vi "日志、报警信息存储 (子VI).vi"() -> ()   [LabVIEW 2016, in "超标留样集成.lvlib" / "德润DR803M超标留样.lvlib"]
uses:
  <vilib>/ptbypt/NI_PtbyPt.lvlib
panel:
  out "MB仪器状态":T1 {"当前进程" items=["停止中"=0, "启动延时"=1, "外置泵延时"=2, "管路润洗"=3, "管存"=4, "留样"=5, "出水管路排空"=6, "采水管路排空"=7, "瓶位调整"=12, "待机"=13]; "工作模式" items=["定时留样"=1, "时间等比"=2, "同步留样"=3, "外控留样"=4, "超标留样"=5]; "仪器时间" format="%<%Y/%m/%d %H:%M:%S>T"}
  out "仪器状态":T2 {"仪器时间" format="%<%Y/%m/%d %H:%M:%S>T"; "门状态" items=["关闭", "打开"]; "采样模式" items=["定时留样"=1, "时间等比"=2, "同步留样"=3, "外控留样"=4, "超标留样"=5]; "工作进程" items=["停止中"=0, "启动延时"=1, "外置泵延时"=2, "管路润洗"=3, "管存"=4, "留样"=5, "出水管路排空"=6, "采水管路排空"=7, "待机"=13]; "工作状态" items=["停止", "运行", "系统初始化"]}
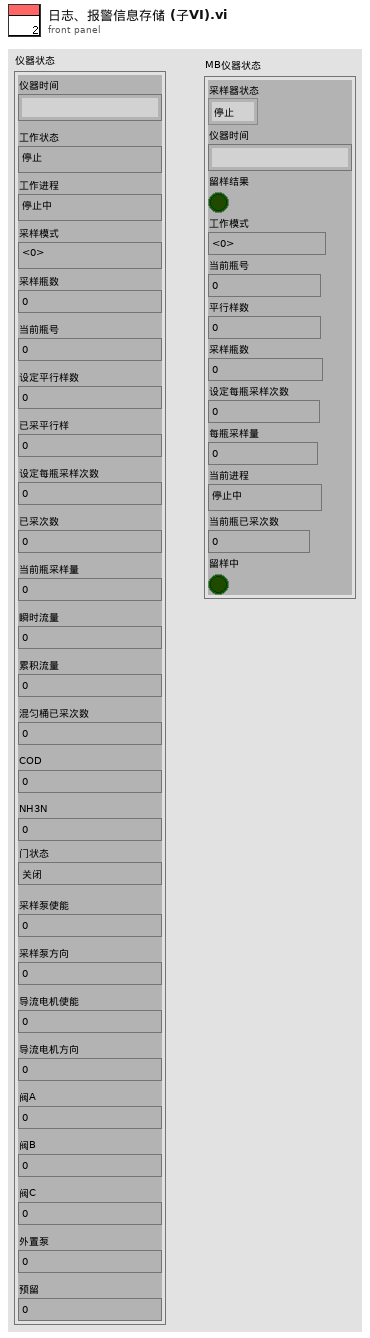
[diagram p1: front panel]
types:
  T1 = cluster{"采样器状态":enum16{"停止", "运行", "系统初始化-2", "系统初始化-3", "初始化失败"}, "仪器时间":timestamp, "留样结果":bool, "工作模式":u16, "当前瓶号":u16, "平行样数":u16, "采样瓶数":u16, "设定每瓶采样次数":u16, "每瓶采样量":u16, "当前进程":u16, "当前瓶已采次数":u16, "留样中":bool}
  T2 = cluster{"仪器时间":timestamp, "工作状态":u16, "工作进程":u16, "采样模式":u16, "采样瓶数":dbl, "当前瓶号":dbl, "设定平行样数":dbl, "已采平行样":dbl, "设定每瓶采样次数":dbl, "已采次数":dbl, "当前瓶采样量":dbl, "瞬时流量":dbl, "累积流量":dbl, "混匀桶已采次数":dbl, "COD":dbl, "NH3N":dbl, "门状态":u16, "采样泵使能":dbl, "采样泵方向":dbl, "导流电机使能":dbl, "导流电机方向":dbl, "阀A":dbl, "阀B":dbl, "阀C":dbl, "外置泵":dbl, "预留":dbl}
  T3 = cluster{"时间标识":timestamp, "设备":string, "日志信息":string}
  T4 = cluster{"时间标识":timestamp, "设备":string, "日志信息":string, "流程参数":string}
  T5 = enum16{"停止", "运行", "系统初始化-2", "系统初始化-3", "初始化失败"}
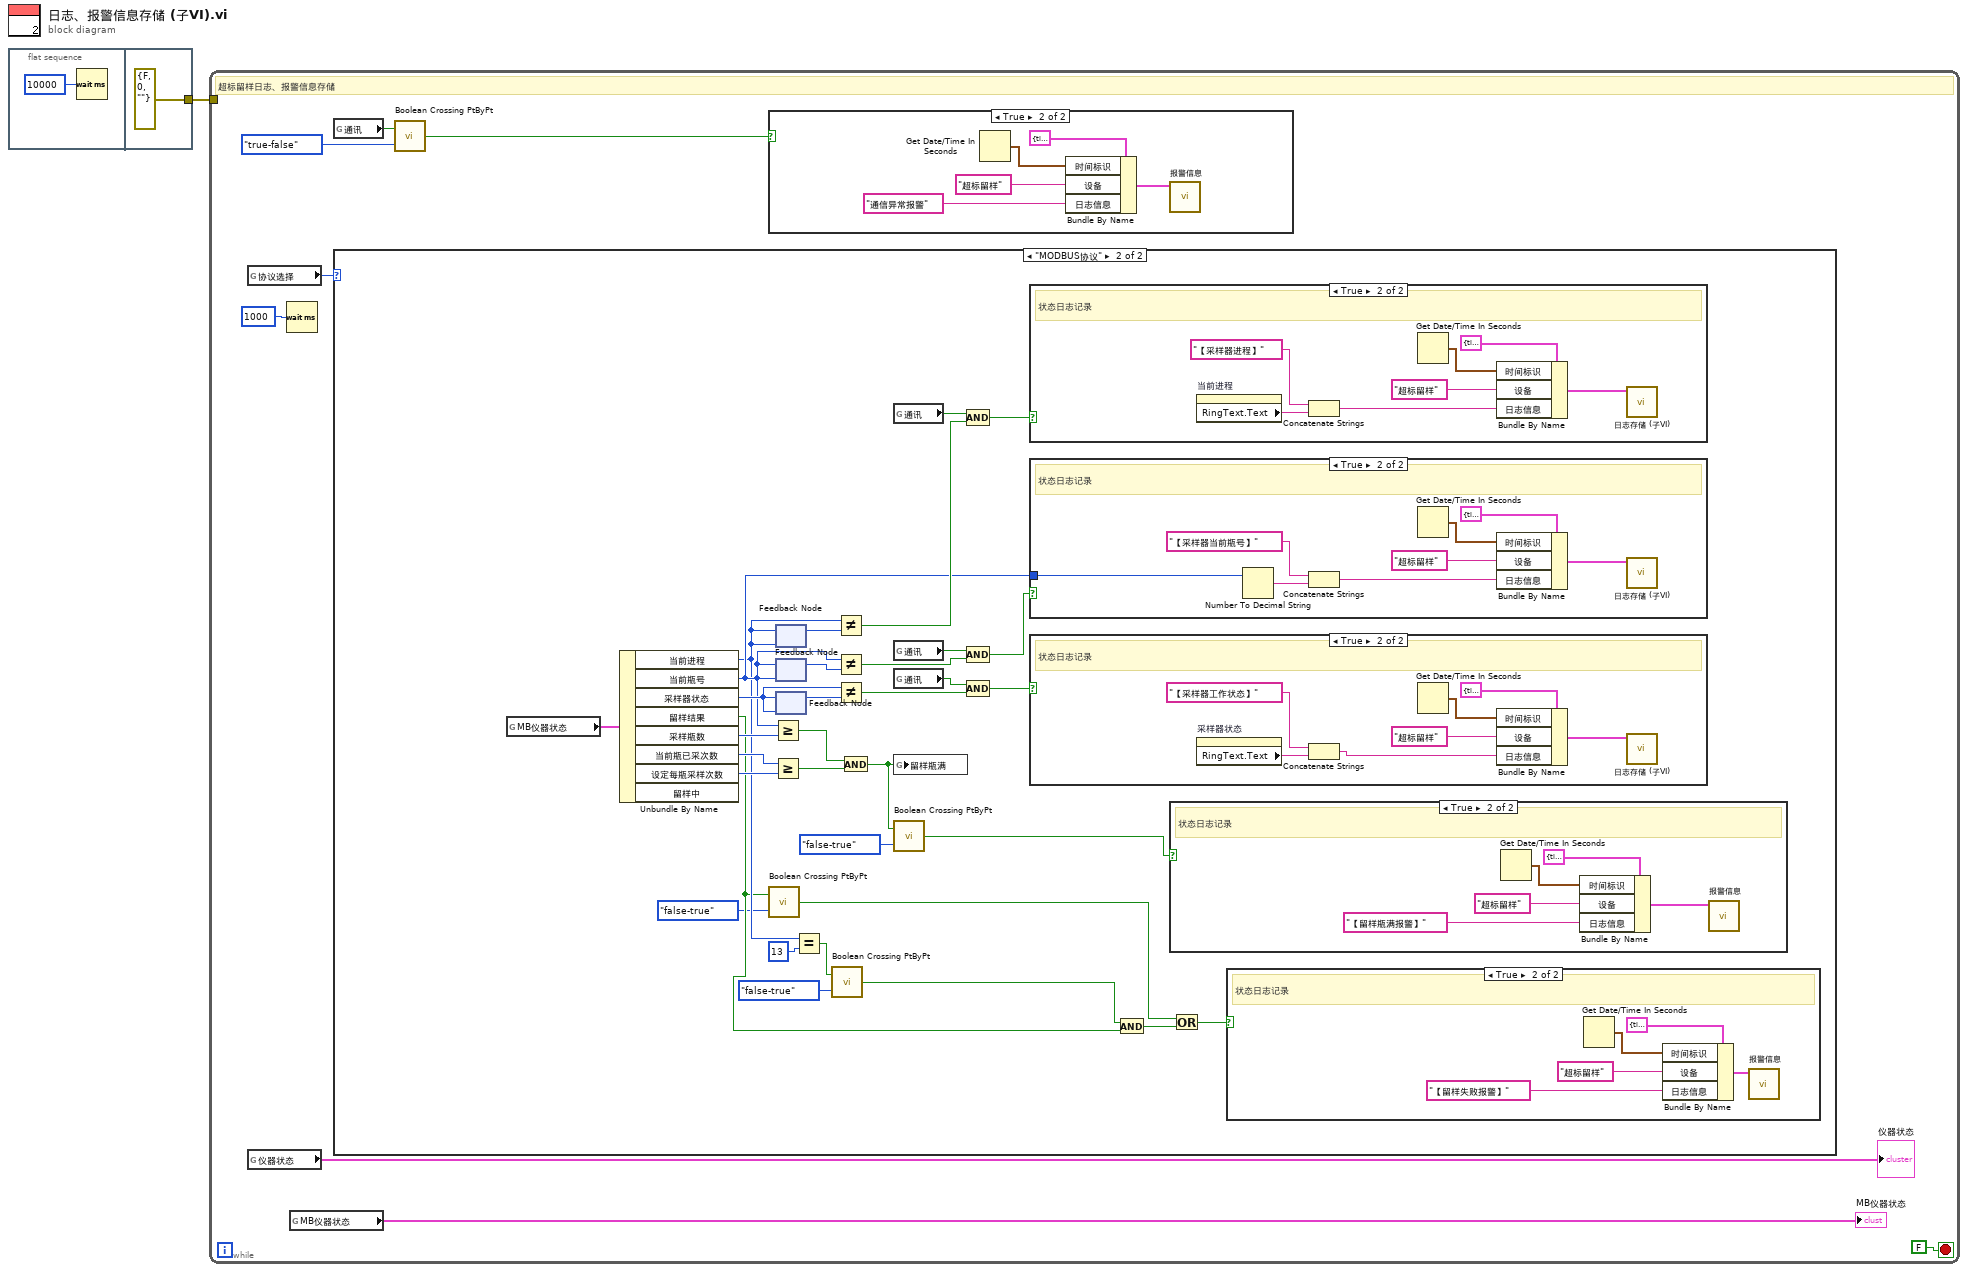
[diagram p0: block diagram]
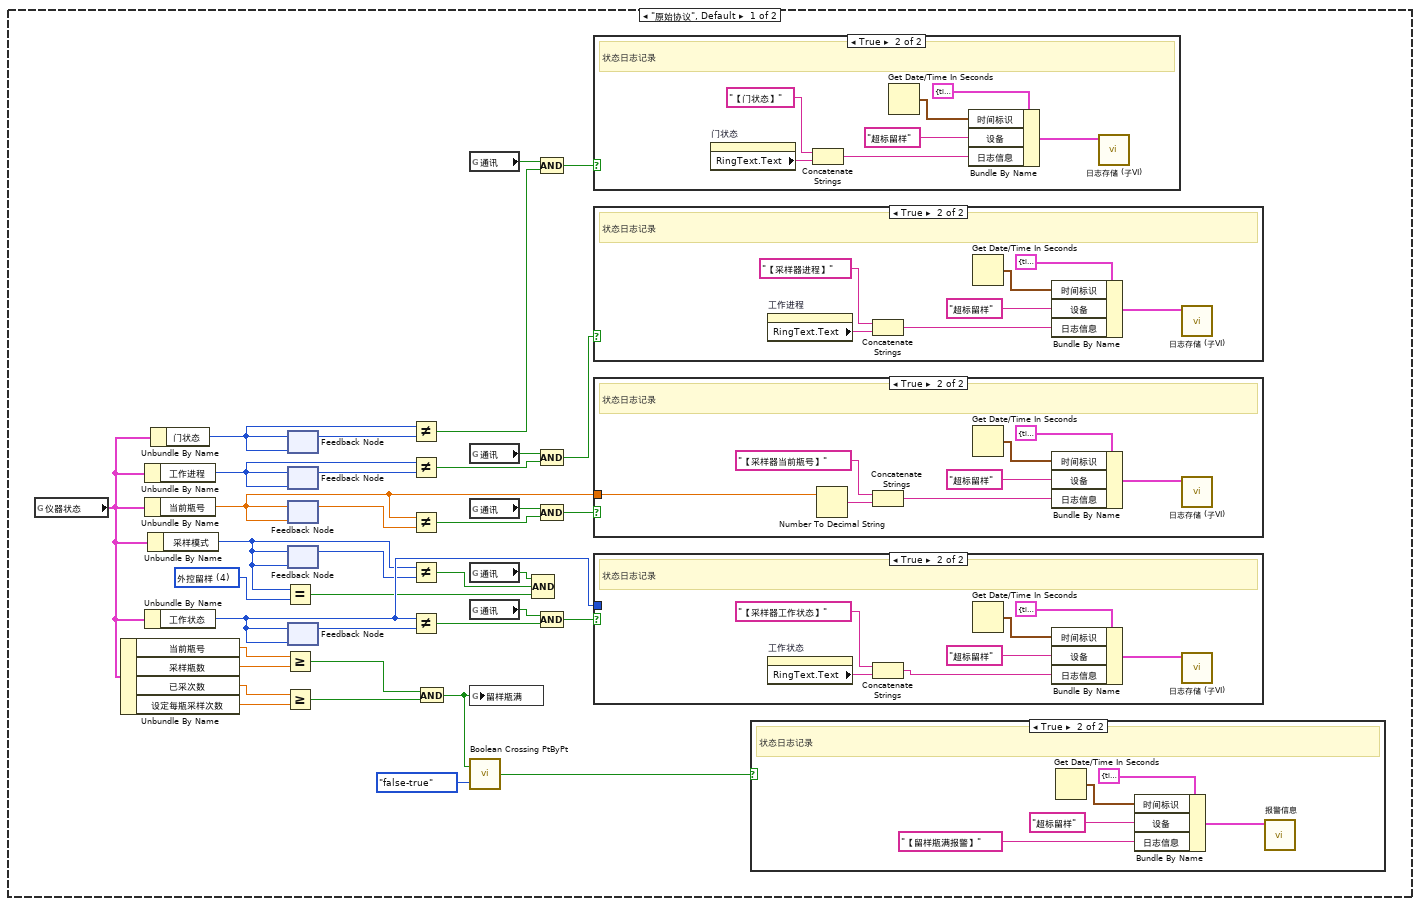
[diagram p2: hidden frame]
diagram:
  n1 = flat-sequence {
    tunnel: [errorcluster {"status"=FALSE, "code"=0, "source"=""} ("错误常量")] -> w1
    frame #0 {
      n2 = Wait (ms)(milliseconds to wait=u32 10000 ("等待时间（毫秒）")) -> ()  [unwired: 1 out]
    }
    frame #1 {
    }
  }
  n3 = while {
    tunnel: w1 -> [_]
    stop <- FALSE stop-if-true
    # "超标留样日志、报警信息存储"
    n4 = global read "超标留样全局.vi" "协议选择"() -> (w6:enum16{"原始协议", "MODBUS协议"})
    n5 = global read "超标留样全局.vi" "仪器状态"() -> (→"仪器状态":T2)
    n6 = Wait (ms)(milliseconds to wait=u32 1000 ("等待时间（毫秒）")) -> ()  [unwired: 1 out]
    n7 = global read "超标留样全局.vi" "MB仪器状态"() -> (→"MB仪器状态":T1)
    n8 = global read "超标留样全局.vi" "通讯"() -> (w7:bool)
    n9 = case shown="\"MODBUS协议\"" w6 {
      frame "原始协议", Default {
        w23 = u16 4 items=["定时留样"=1, "时间等比"=2, "同步留样"=3, "外控留样"=4, "超标留样"=5] ("采样模式")
        n10 = global read "超标留样全局.vi" "仪器状态"() -> (w22:T2)
        n11 = Unbundle By Name(w22) -> ("当前瓶号"=w21:dbl, "采样瓶数"=w20:dbl, "已采次数"=w19:dbl, "设定每瓶采样次数"=w18:dbl)
        n12 = Unbundle By Name(w22) -> ("工作进程"=w47:u16)
        n13 = Unbundle By Name(w22) -> ("当前瓶号"=w44:dbl)
        n14 = Unbundle By Name(w22) -> ("工作状态"=w43:u16)
        n15 = Unbundle By Name(w22) -> ("采样模式"=w39:u16)
        n16 = Unbundle By Name(w22) -> ("门状态"=w40:u16)
        n17 = Equal?(x=w39, y=w23) -> (x = y?=w25:bool)
        n18 = Greater Or Equal?(x=w21, y=w20) -> (x >= y?=w17:bool)
        n19 = Greater Or Equal?(x=w19, y=w18) -> (x >= y?=w16:bool)
        n20 = feedback #1(w40) -> (w41:u16)
        n21 = feedback-in #1(w40) -> ()
        n22 = feedback #2(w47) -> (w46:u16)
        n23 = feedback-in #2(w47) -> ()
        n24 = feedback #3(w44) -> (w45:dbl)
        n25 = feedback-in #3(w44) -> ()
        n26 = feedback #4(w39) -> (w38:u16)
        n27 = feedback-in #4(w39) -> ()
        n28 = feedback #5(w43) -> (w42:u16)
        n29 = feedback-in #5(w43) -> ()
        n30 = Not Equal?(x=w40, y=w41) -> (x != y?=w35:bool)
        n31 = Not Equal?(x=w47, y=w46) -> (x != y?=w33:bool)
        n32 = Not Equal?(x=w44, y=w45) -> (x != y?=w30:bool)
        n33 = Not Equal?(x=w39, y=w38) -> (x != y?=w24:bool)
        n34 = Not Equal?(x=w43, y=w42) -> (x != y?=w28:bool)
        n35 = And(x=w17, y=w16) -> (x .and. y?=w13:bool)
        n36 = global read "超标留样全局.vi" "通讯"() -> (w37:bool)
        n37 = global read "超标留样全局.vi" "通讯"() -> (w34:bool)
        n38 = global read "超标留样全局.vi" "通讯"() -> (w32:bool)
        n39 = global read "超标留样全局.vi" "通讯"() -> (w26:bool)
        n40 = global read "超标留样全局.vi" "通讯"() -> (w29:bool)
        n41 = global write "超标留样全局.vi" "留样瓶满"(w13) -> ()
        n42 = call <vilib>:"Boolean Crossing PtByPt.vi"("direction"=enum16{"either", "false-true", "true-false"}."false-true", "input"=w13) -> ("crossing"=w14:bool)  [unwired: 1 in]
        n43 = Compound Arithmetic op=AND ("复合运算")(w26, w24, w25) -> ()  [unwired: 1 out]
        n44 = Compound Arithmetic op=AND ("复合运算")(w37, w35) -> (w36:bool)
        n45 = Compound Arithmetic op=AND ("复合运算")(w34, w33) -> (w12:bool)
        n46 = Compound Arithmetic op=AND ("复合运算")(w32, w30) -> (w31:bool)
        n47 = Compound Arithmetic op=AND ("复合运算")(w29, w28) -> (w27:bool)
        n48 = case shown="True" w36 {
          frame False {
          }
          frame True {
            # "状态日志记录"
            n49 = property on="门状态" class="Ring (strict)"() -> ("RingText.Text"=w53:string)  [unwired: 2 in, 2 out]
            n50 = Concatenate Strings("【门状态】" ("日志信息"), w53) -> (w59:string)
            n51 = Get Date/Time In Seconds() -> (seconds since 1Jan1904=w56:timestamp)
            n52 = Bundle By Name(cluster=T4 {"时间标识"=timestamp(0 s since 1904-01-01), "设备"="", "日志信息"="", "流程参数"=""} ("data in"), "时间标识"=w56, "设备"="超标留样", "日志信息"=w59) -> (w55:T4)
            n53 = call "日志存储 (子VI).vi"("data in"=w55) -> ()  [unwired: 11 in]
          }
        }
        n54 = case shown="True" w12 {
          frame False {
          }
          frame True {
            # "状态日志记录"
            n55 = property on="工作进程" class="Ring (strict)"() -> ("RingText.Text"=w75:string)  [unwired: 2 in, 2 out]
            n56 = Concatenate Strings("【采样器进程】" ("日志信息"), w75) -> (w81:string)
            n57 = Get Date/Time In Seconds() -> (seconds since 1Jan1904=w78:timestamp)
            n58 = Bundle By Name(cluster=T4 {"时间标识"=timestamp(0 s since 1904-01-01), "设备"="", "日志信息"="", "流程参数"=""} ("data in"), "时间标识"=w78, "设备"="超标留样", "日志信息"=w81) -> (w77:T4)
            n59 = call "日志存储 (子VI).vi"("data in"=w77) -> ()  [unwired: 11 in]
          }
        }
        n60 = case shown="True" w31 {
          tunnel: w44 -> [_ w68]
          frame False {
          }
          frame True {
            # "状态日志记录"
            n61 = Number To Decimal String(number=w68) -> (decimal integer string=w67:string)  [unwired: 1 in]
            n62 = Concatenate Strings("【采样器当前瓶号】" ("日志信息"), w67) -> (w74:string)
            n63 = Get Date/Time In Seconds() -> (seconds since 1Jan1904=w71:timestamp)
            n64 = Bundle By Name(cluster=T4 {"时间标识"=timestamp(0 s since 1904-01-01), "设备"="", "日志信息"="", "流程参数"=""} ("data in"), "时间标识"=w71, "设备"="超标留样", "日志信息"=w74) -> (w70:T4)
            n65 = call "日志存储 (子VI).vi"("data in"=w70) -> ()  [unwired: 11 in]
          }
        }
        n66 = case shown="True" w27 {
          tunnel: w43 -> [_ _]
          frame False {
          }
          frame True {
            # "状态日志记录"
            n67 = property on="工作状态" class="Ring (strict)"() -> ("RingText.Text"=w60:string)  [unwired: 2 in, 2 out]
            n68 = Concatenate Strings("【采样器工作状态】" ("日志信息"), w60) -> (w66:string)
            n69 = Get Date/Time In Seconds() -> (seconds since 1Jan1904=w63:timestamp)
            n70 = Bundle By Name(cluster=T4 {"时间标识"=timestamp(0 s since 1904-01-01), "设备"="", "日志信息"="", "流程参数"=""} ("data in"), "时间标识"=w63, "设备"="超标留样", "日志信息"=w66) -> (w62:T4)
            n71 = call "日志存储 (子VI).vi"("data in"=w62) -> ()  [unwired: 11 in]
          }
        }
        n72 = case shown="True" w14 {
          frame False {
          }
          frame True {
            # "状态日志记录"
            n73 = Get Date/Time In Seconds() -> (seconds since 1Jan1904=w51:timestamp)
            n74 = Bundle By Name(cluster=T3 {"时间标识"=timestamp(0 s since 1904-01-01), "设备"="", "日志信息"=""} ("data in"), "时间标识"=w51, "设备"="超标留样", "日志信息"="【留样瓶满报警】") -> (w49:T3)
            n75 = call "报警信息.vi"("data in"=w49) -> ()  [unwired: 10 in, 1 out]
          }
        }
      }
      frame "MODBUS协议" {
        n76 = global read "超标留样全局.vi" "MB仪器状态"() -> (w100:T1)
        n77 = Unbundle By Name(w100) -> ("当前进程"=w88:u16, "当前瓶号"=w97:u16, "采样器状态"=w112:T5, "留样结果"=w84:bool, "采样瓶数"=w96:u16, "当前瓶已采次数"=w95:u16, "设定每瓶采样次数"=w94:u16)  [unwired: 1 out]
        n78 = call <vilib>:"Boolean Crossing PtByPt.vi"("direction"=enum16{"either", "false-true", "true-false"}."false-true", "input"=w84) -> ("crossing"=w82:bool)  [unwired: 1 in]
        n79 = Greater Or Equal?(x=w97, y=w96) -> (x >= y?=w99:bool)
        n80 = Greater Or Equal?(x=w95, y=w94) -> (x >= y?=w98:bool)
        n81 = feedback #6(w88) -> (w101:u16)
        n82 = feedback-in #6(w88) -> ()
        n83 = feedback #7(w97) -> (w104:u16)
        n84 = feedback-in #7(w97) -> ()
        n85 = feedback #8(w112) -> (w111:T5)
        n86 = feedback-in #8(w112) -> ()
        n87 = Equal?(x=w88, y=u16 13) -> (x = y?=w86:bool)
        n88 = call <vilib>:"Boolean Crossing PtByPt.vi"("direction"=enum16{"either", "false-true", "true-false"}."false-true", "input"=w86) -> ("crossing"=w85:bool)  [unwired: 1 in]
        n89 = Not Equal?(x=w88, y=w101) -> (x != y?=w103:bool)
        n90 = Not Equal?(x=w97, y=w104) -> (x != y?=w106:bool)
        n91 = Not Equal?(x=w112, y=w111) -> (x != y?=w109:bool)
        n92 = And(x=w99, y=w98) -> (x .and. y?=w91:bool)
        n93 = global read "超标留样全局.vi" "通讯"() -> (w102:bool)
        n94 = global read "超标留样全局.vi" "通讯"() -> (w105:bool)
        n95 = global read "超标留样全局.vi" "通讯"() -> (w110:bool)
        n96 = global write "超标留样全局.vi" "留样瓶满"(w91) -> ()
        n97 = call <vilib>:"Boolean Crossing PtByPt.vi"("direction"=enum16{"either", "false-true", "true-false"}."false-true", "input"=w91) -> ("crossing"=w92:bool)  [unwired: 1 in]
        n98 = Compound Arithmetic op=AND ("复合运算")(w102, w103) -> (w108:bool)
        n99 = Compound Arithmetic op=AND ("复合运算")(w105, w106) -> (w107:bool)
        n100 = Compound Arithmetic op=AND ("复合运算")(w110, w109) -> (w113:bool)
        n101 = case shown="True" w108 {
          frame False {
          }
          frame True {
            # "状态日志记录"
            n102 = property on="当前进程" class="Ring (strict)"() -> ("RingText.Text"=w140:string)  [unwired: 2 in, 2 out]
            n103 = Concatenate Strings("【采样器进程】" ("日志信息"), w140) -> (w146:string)
            n104 = Get Date/Time In Seconds() -> (seconds since 1Jan1904=w143:timestamp)
            n105 = Bundle By Name(cluster=T4 {"时间标识"=timestamp(0 s since 1904-01-01), "设备"="", "日志信息"="", "流程参数"=""} ("data in"), "时间标识"=w143, "设备"="超标留样", "日志信息"=w146) -> (w142:T4)
            n106 = call "日志存储 (子VI).vi"("data in"=w142) -> ()  [unwired: 11 in]
          }
        }
        n107 = case shown="True" w107 {
          tunnel: w97 -> [_ w133]
          frame False {
          }
          frame True {
            # "状态日志记录"
            n108 = Number To Decimal String(number=w133) -> (decimal integer string=w132:string)  [unwired: 1 in]
            n109 = Concatenate Strings("【采样器当前瓶号】" ("日志信息"), w132) -> (w139:string)
            n110 = Get Date/Time In Seconds() -> (seconds since 1Jan1904=w136:timestamp)
            n111 = Bundle By Name(cluster=T4 {"时间标识"=timestamp(0 s since 1904-01-01), "设备"="", "日志信息"="", "流程参数"=""} ("data in"), "时间标识"=w136, "设备"="超标留样", "日志信息"=w139) -> (w135:T4)
            n112 = call "日志存储 (子VI).vi"("data in"=w135) -> ()  [unwired: 11 in]
          }
        }
        n113 = case shown="True" w113 {
          frame False {
          }
          frame True {
            # "状态日志记录"
            n114 = property on="采样器状态" class="Enum (strict)"() -> ("RingText.Text"=w125:string)  [unwired: 2 in, 2 out]
            n115 = Concatenate Strings("【采样器工作状态】" ("日志信息"), w125) -> (w131:string)
            n116 = Get Date/Time In Seconds() -> (seconds since 1Jan1904=w128:timestamp)
            n117 = Bundle By Name(cluster=T4 {"时间标识"=timestamp(0 s since 1904-01-01), "设备"="", "日志信息"="", "流程参数"=""} ("data in"), "时间标识"=w128, "设备"="超标留样", "日志信息"=w131) -> (w127:T4)
            n118 = call "日志存储 (子VI).vi"("data in"=w127) -> ()  [unwired: 11 in]
          }
        }
        n119 = And(x=w85, y=w84) -> (x .and. y?=w89:bool)
        n120 = case shown="True" w92 {
          frame False {
          }
          frame True {
            # "状态日志记录"
            n121 = Get Date/Time In Seconds() -> (seconds since 1Jan1904=w118:timestamp)
            n122 = Bundle By Name(cluster=T3 {"时间标识"=timestamp(0 s since 1904-01-01), "设备"="", "日志信息"=""} ("data in"), "时间标识"=w118, "设备"="超标留样", "日志信息"="【留样瓶满报警】") -> (w116:T3)
            n123 = call "报警信息.vi"("data in"=w116) -> ()  [unwired: 10 in, 1 out]
          }
        }
        n124 = Or(x=w82, y=w89) -> (x .or. y?=w90:bool)
        n125 = case shown="True" w90 {
          frame False {
          }
          frame True {
            # "状态日志记录"
            n126 = Get Date/Time In Seconds() -> (seconds since 1Jan1904=w123:timestamp)
            n127 = Bundle By Name(cluster=T3 {"时间标识"=timestamp(0 s since 1904-01-01), "设备"="", "日志信息"=""} ("data in"), "时间标识"=w123, "设备"="超标留样", "日志信息"="【留样失败报警】") -> (w121:T3)
            n128 = call "报警信息.vi"("data in"=w121) -> ()  [unwired: 10 in, 1 out]
          }
        }
      }
    }
    n129 = call <vilib>:"Boolean Crossing PtByPt.vi"("direction"=enum16{"either", "false-true", "true-false"}."true-false", "input"=w7) -> ("crossing"=w8:bool)  [unwired: 1 in]
    n130 = case shown="True" w8 {
      frame False {
      }
      frame True {
        n131 = Get Date/Time In Seconds() -> (seconds since 1Jan1904=w148:timestamp)
        n132 = Bundle By Name(cluster=T3 {"时间标识"=timestamp(0 s since 1904-01-01), "设备"="", "日志信息"=""} ("data in"), "时间标识"=w148, "设备"="超标留样", "日志信息"="通信异常报警") -> (w147:T3)
        n133 = call "报警信息.vi"("data in"=w147) -> ()  [unwired: 10 in, 1 out]
      }
    }
  }
